vi "Exit.vi"(8 "error in (no error)":errorcluster, 11 "Old State":refnum<class "GTH-Down.lvclass">) -> (0 "error out":errorcluster, 3 "New State":refnum<class "GTH-Down.lvclass">)   [LabVIEW 2014, in "Elevator.lvlib" / "EL-Go To Height.lvlib" / "GTH-Down.lvclass"]
doc: "This is an abstract method. Override this method to define the behavior when you leave the state."
uses:
  GTH-Down.lvclass
  Elevator Messages/Set Rate (Percent) Msg/Set Rate (Percent) Msg.lvclass/Set Rate (Percent) Msg.ctl
  <vilib>/ActorFramework/Message Enqueuer/Message Enqueuer.lvclass/Message Enqueuer.ctl
  <vilib>/ActorFramework/Message Enqueuer/Enqueue.vi
  <vilib>/ActorFramework/Message Priority Queue/Priority Enqueue.vi
  Elevator Messages/Set Rate (Percent) Msg/Set Rate (Percent) Msg.lvclass
  EL-Go To Height Class/EL-Go To Height.lvclass
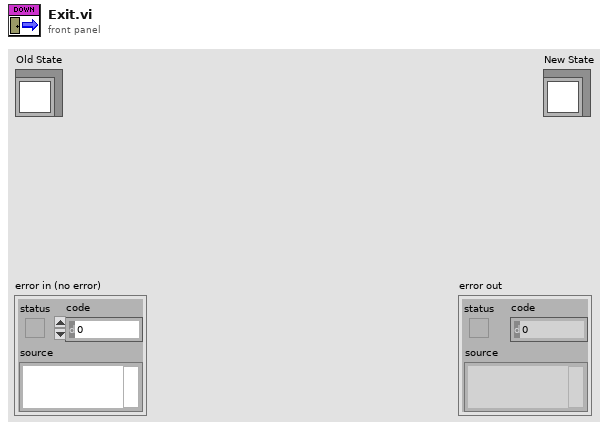
[diagram p1: front panel]
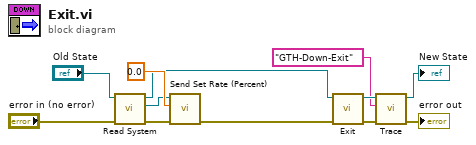
[diagram p0: block diagram]
diagram:
  n1 = call-dynamic "Read System.vi"("error in (no error)"="error in (no error)", "Command in"="Old State") -> ("error out"=w11:errorcluster, "Actor Framework:Message Enqueuer"=w9:refnum<class "Message Enqueuer.lvclass">, "Command out"=w8:refnum<class "GTH-Down.lvclass">)  [unwired: 7 in]
  n2 = call "Send Set Rate (Percent).vi"("error in (no error)"=w11, "Percent"=0.0, "Message Enqueuer"=w9) -> ("error out"=w4:errorcluster)  [unwired: 7 in, 1 out]
  n3 = call-parent "Exit.vi"("error in (no error)"=w4, "Old State"=w8) -> ("error out"=w3:errorcluster, "New State"=w6:refnum<class "GTH-Down.lvclass">)  [unwired: 8 in]
  n4 = call-dynamic "Trace.vi"("error in (no error)"=w3, "Command Action"="GTH-Down-Exit", "Command Actor in"=w6) -> ("error out"=→"error out":errorcluster, "Command Actor out"=→"New State":refnum<class "GTH-Down.lvclass">)  [unwired: 7 in]
